vi "Write Addend 1.vi"(8 "error in (no error)":errorcluster, 10 "Addend 1":dbl, 11 "SimpleAdder in":refnum<class "SimpleAdder.lvclass">) -> (0 "error out":errorcluster, 3 "SimpleAdder out":refnum<class "SimpleAdder.lvclass">)   [LabVIEW 2012, in "SimpleAdder.lvclass"]
uses:
  SimpleAdder.lvclass
  SimpleAdder.lvclass/SimpleAdder.ctl
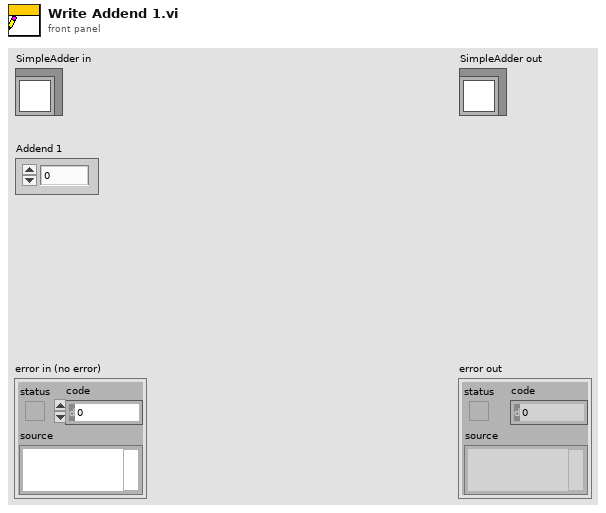
[diagram p1: front panel]
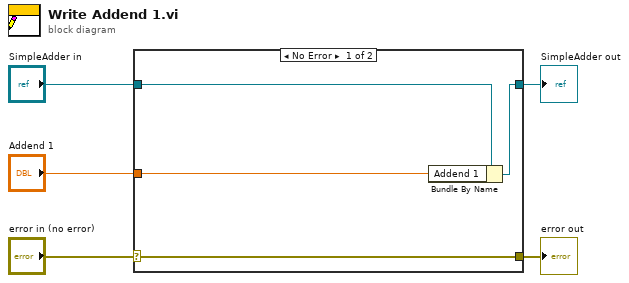
[diagram p0: block diagram]
diagram:
  n1 = case shown="No Error" "error in (no error)" {
    selector: "error in (no error)" -> [w9 w10]
    tunnel: [w9 w10] -> w4
    tunnel: [w7 w11] -> w2
    tunnel: "SimpleAdder in" -> [w8 w11]
    tunnel: "Addend 1" -> [w6 _]
    frame No Error {
      n2 = Bundle By Name(cluster=w8, "Addend 1"=w6) -> (w7:refnum<class "SimpleAdder.lvclass">)
    }
    frame Error {
    }
  }
  "error out" <- w4
  "SimpleAdder out" <- w2
